vi "Perform Action.vi"(8 "error in":errorcluster, 10 "Input":variant, 11 "AO DAQmx DC Simulated CFG in":refnum<class "AO DAQmx DC CFG Simulated.lvclass">) -> (0 "error out":errorcluster, 2 "Output":variant, 3 "AO DAQmx DC Simulated CFG out":refnum<class "AO DAQmx DC CFG Simulated.lvclass">)   [LabVIEW 2024, in "DAQmx Simulated CFGs.lvlib" / "AO DAQmx DC CFG Simulated.lvclass"]
uses:
  AO DAQmx DC CFG Simulated.lvclass
  AO DAQmx DC CFG/AO DAQmx DC CFG.lvclass
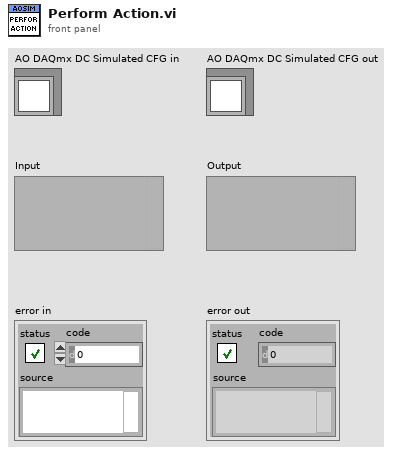
[diagram p1: front panel]
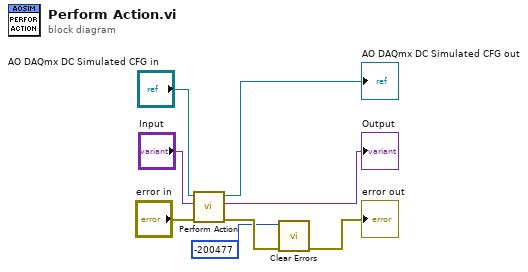
[diagram p0: block diagram]
diagram:
  n1 = call-parent "Perform Action.vi"("error in"="error in", "Input"="Input", "AO DAQmx DC CFG in"="AO DAQmx DC Simulated CFG in") -> ("error out"=w8:errorcluster, "Output"=→"Output":variant, "AO DAQmx DC CFG out"=→"AO DAQmx DC Simulated CFG out":refnum<class "AO DAQmx DC CFG Simulated.lvclass">)  [unwired: 6 in]
  n2 = call <vilib>:"Clear Errors.vi"("error in (no error)"=w8, "specific error code to clear (0: all)"=-200477) -> ("error out"=→"error out":errorcluster)  [unwired: 4 in, 1 out]
